vi "ProceListActMain.vi"() -> ()   [LabVIEW 2019]
uses:
  Ctrl/Right2arrow.ctl
  Ctrl/left2arrow.ctl
  Ctrl/UpLoad2.ctl
  Ctrl/Remove.ctl
  Ctrl/Up2.ctl
  Ctrl/down2.ctl
  <vilib>/Utility/miscctls.llb/LVPointTypeDef.ctl
  <vilib>/Utility/miscctls.llb/LVPositionTypeDef.ctl
  60868002-0d4d-43f0-995a-60bbf307d005.vi
  3149b30a-55dc-446c-b552-6eeb82815ac3.vi
  963f54ab-7a83-4128-af58-6966ad4c5d0f.vi
  27abb3d3-4d96-49e0-85aa-55843c44cf8e.vi
  5b1c7a0c-b8ed-4af5-97c9-577675ba5e56.vi
  577cd01a-d66b-4b05-b2ca-c7f6d430580f.vi
  87e15d9e-a7ef-48ad-a0c8-dc216d43436b.vi
  40c5cbea-e99d-4875-be97-d34c3ca007e7.vi
  <vilib>/JDP Science/JSONtext/JSON text to Variant.vi
  LLB/Commonly VI/Main Glb.vi
  Glb/ProcessListGlb.vi
  Class/Main Process Class/MPC_VirbVision/Panel RefGlb.vi
  <vilib>/JDP Science/JSONtext/Variant to JSON Text.vi
  LLB/Commonly VI.lvlib
panel:
  out "DataOutResult":string caption="輸出資料數據範例"
  out "DataOutName":string caption="輸出資料名稱"
  in  "SelectUp":T1
  in  "SelectDown":T2
  out "Action 2":string
  out "ProceListPath":path
  in  "SubUI":bool
  in  "Tab Control":enum32{"Page 1", "Page 2"}(tab)
  in  "VisionTable":i32(listbox) caption="視覺列表/VisionList"
  in  "Action":enum16{"Vision", "Virbration", "IO"}(ring)=enum."Virbration"
  in  "ProcessPage":T3(tab)=enum."None"
  in  "VisionProjectList":u16(ring) caption="專案選擇/Project Select" items=["None", "Calib", "Check", "Item1", "Item2", "Item3"]
  in  "Btn_AddVirbListAct":T4
  in  "Btn_RemoveVirbListAct":T5
  in  "VirbList":i32(listbox) caption="列表"
  in  "VirbrationProjectList":i32(listbox) caption="專案清單"
  in  "Btn_AddIOListAct":T4
  in  "Btn_RemoveIOListAct":T5
  in  "IOList":i32(listbox) caption="列表"
  in  "IOProjectList":i32(listbox) caption="專案清單"
  in  "VisionCheck":u16(ring) caption="專案選擇/Project Select" items=["None", "Calib", "Check", "Item1", "Item2", "Item3"]
  in  "ActionTable":i32(listbox) caption="動作列表/ActionList"
  in  "InsertToList":T6
  in  "UpdateActLisrVir":bool
  in  "RemoveFroimList":T7
  in  "Btn_Save":bool
  # "請選擇使用定位功能之視覺專案!!!\nPlease Select Vision Project With Location  !!!"
  # "請選擇使用Area Check演算法之視覺專案!!!\nPlease Select Vision Project With Area Check  !!!"
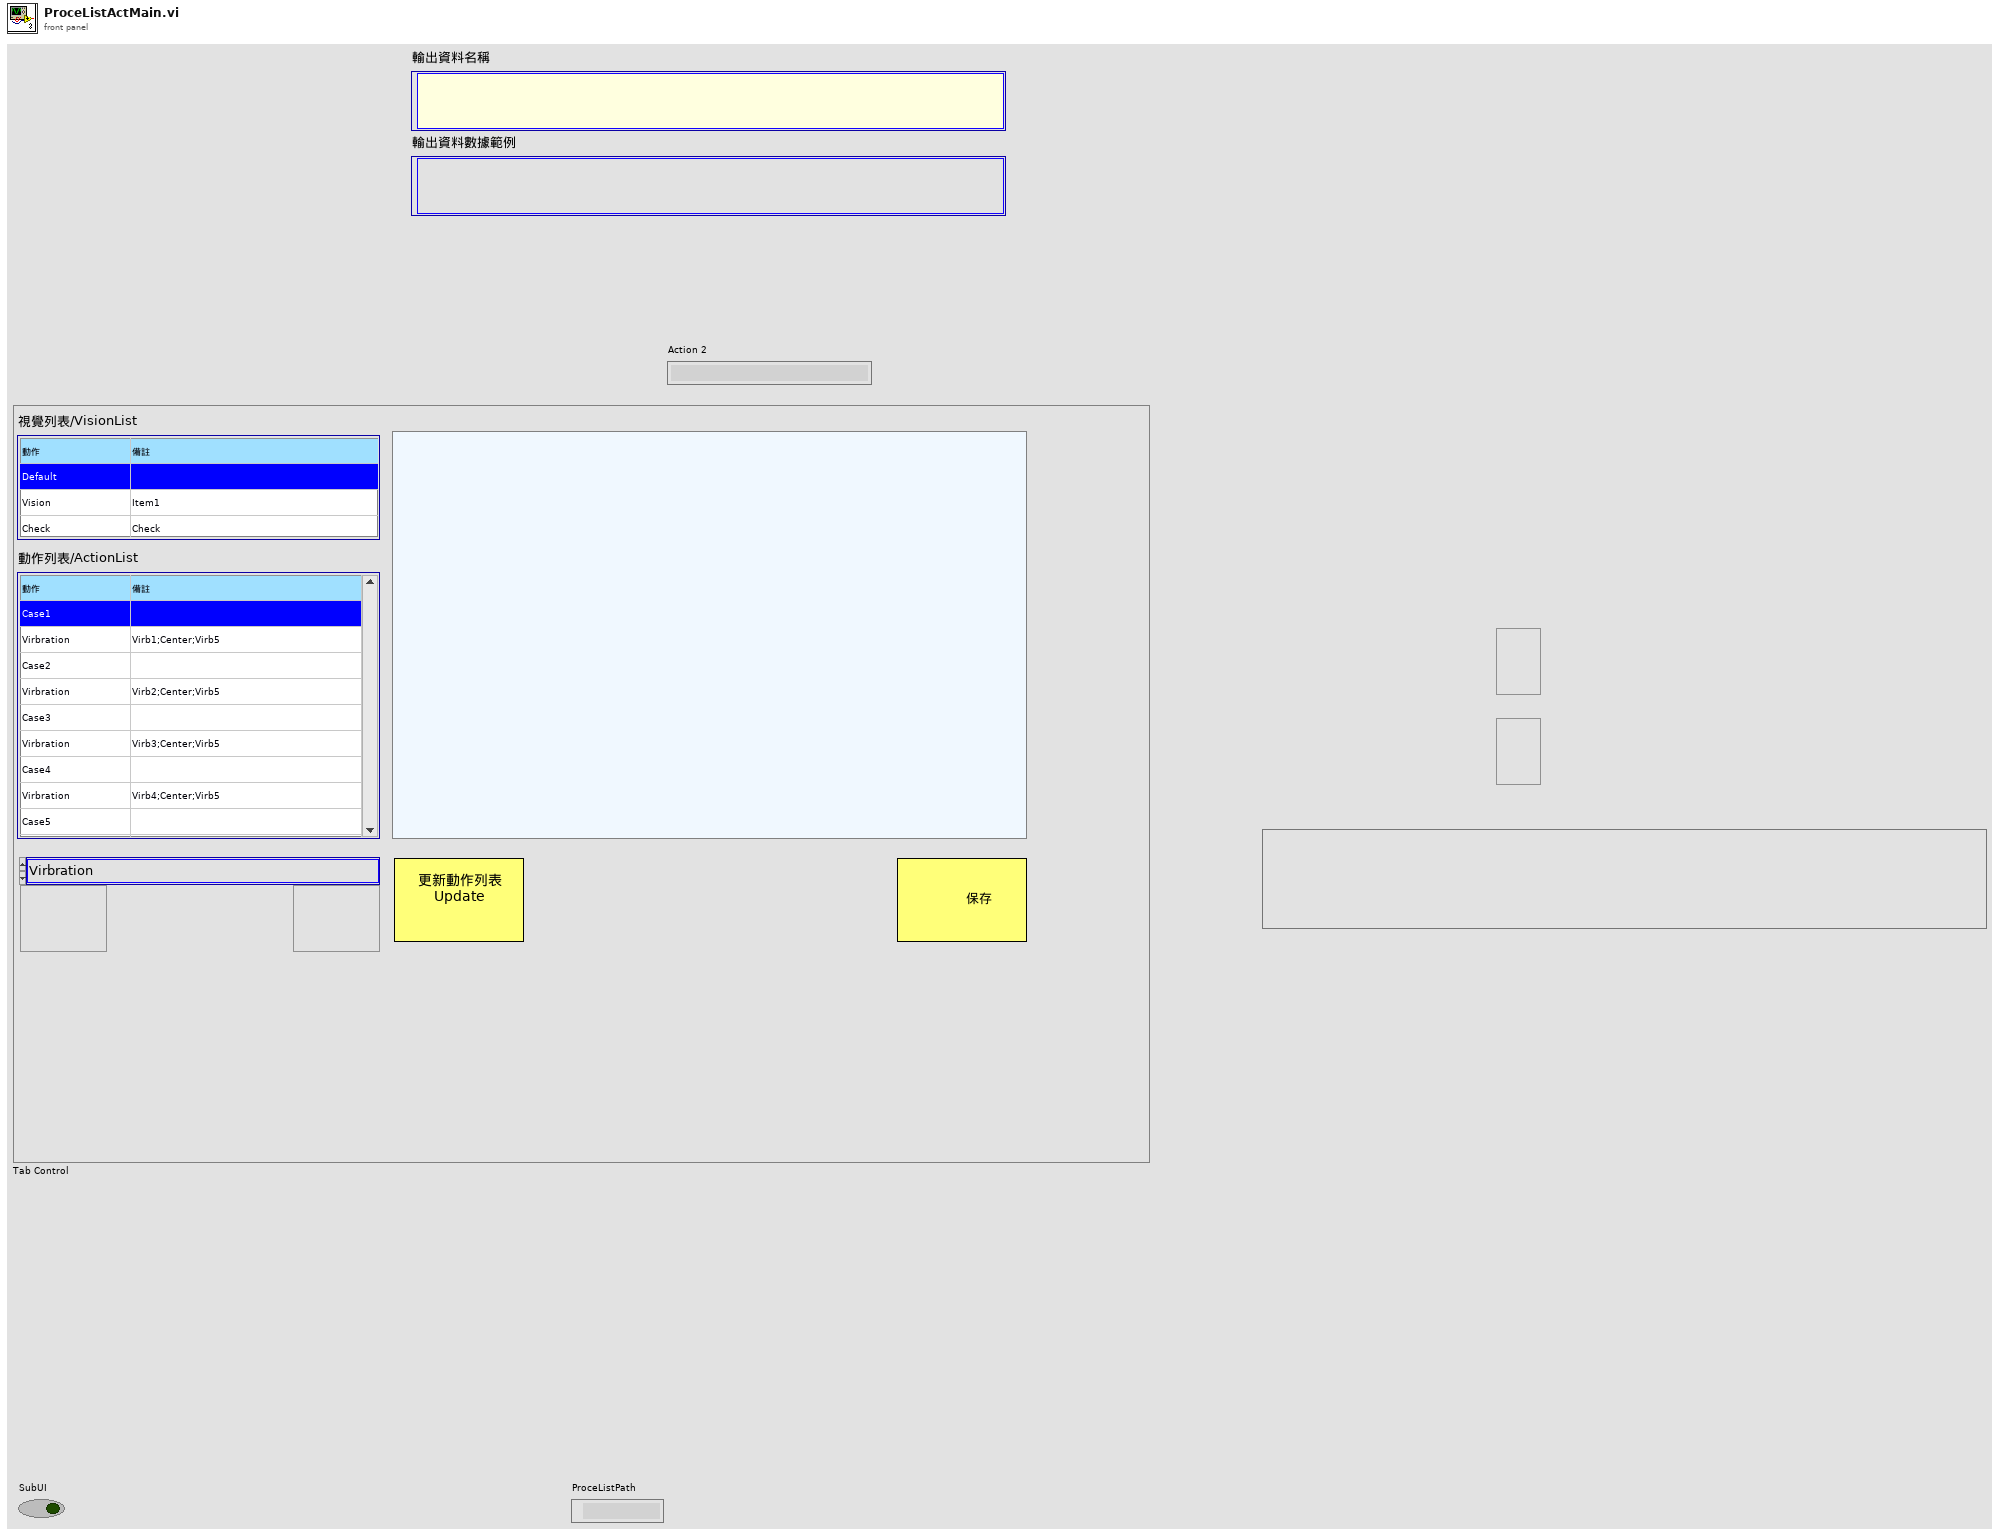
[diagram p1: front panel]
types:
  T1 = typedef "Up2.ctl" = bool
  T2 = typedef "down2.ctl" = bool
  T3 = enum32{"Vision", "Virbration", "IO", "Check", "None"}
  T4 = typedef "Right2arrow.ctl" = bool
  T5 = typedef "left2arrow.ctl" = bool
  T6 = typedef "UpLoad2.ctl" = bool
  T7 = typedef "Remove.ctl" = bool
  T8 = typedef "LVPositionTypeDef.ctl" = cluster{"Left":i32, "Top":i32}
  T9 = typedef "LVPointTypeDef.ctl" = cluster{"Horizontal":i16, "Vertical":i16}
  T10 = enum16{"Initial", "Write", "Read", "Save", "Load", "WrteAll"}
  T11 = enum16{"Initial", "Write", "Read", "Save", "Load", "Add", "Delete"}
  T12 = enum16{"initial", "write", "add", "delete", "Load", "Save", "Read", "ReadProjectName"}
  T13 = cluster{"VirbrationProjectList":refnum<vi>, "OutList":refnum<vi>}
  T14 = enum32{"invalid app kind", "Development System", "Run Time System", "Student Edition", "Embedded LabVIEW", "Evaluation", "Custom"}
  T15 = cluster{"VirbSeqName":string, "VirbSeqStep":string[]}[]
  T16 = typedef "LVPoint32TypeDef.ctl" = cluster{"Horizontal":i32, "Vertical":i32}
  T17 = cluster{"VirbrationProjectList":refnum<vi>, "VirbList":refnum<vi>}
  T18 = cluster{"IOProjectList":refnum<vi>, "IOList":refnum<vi>}
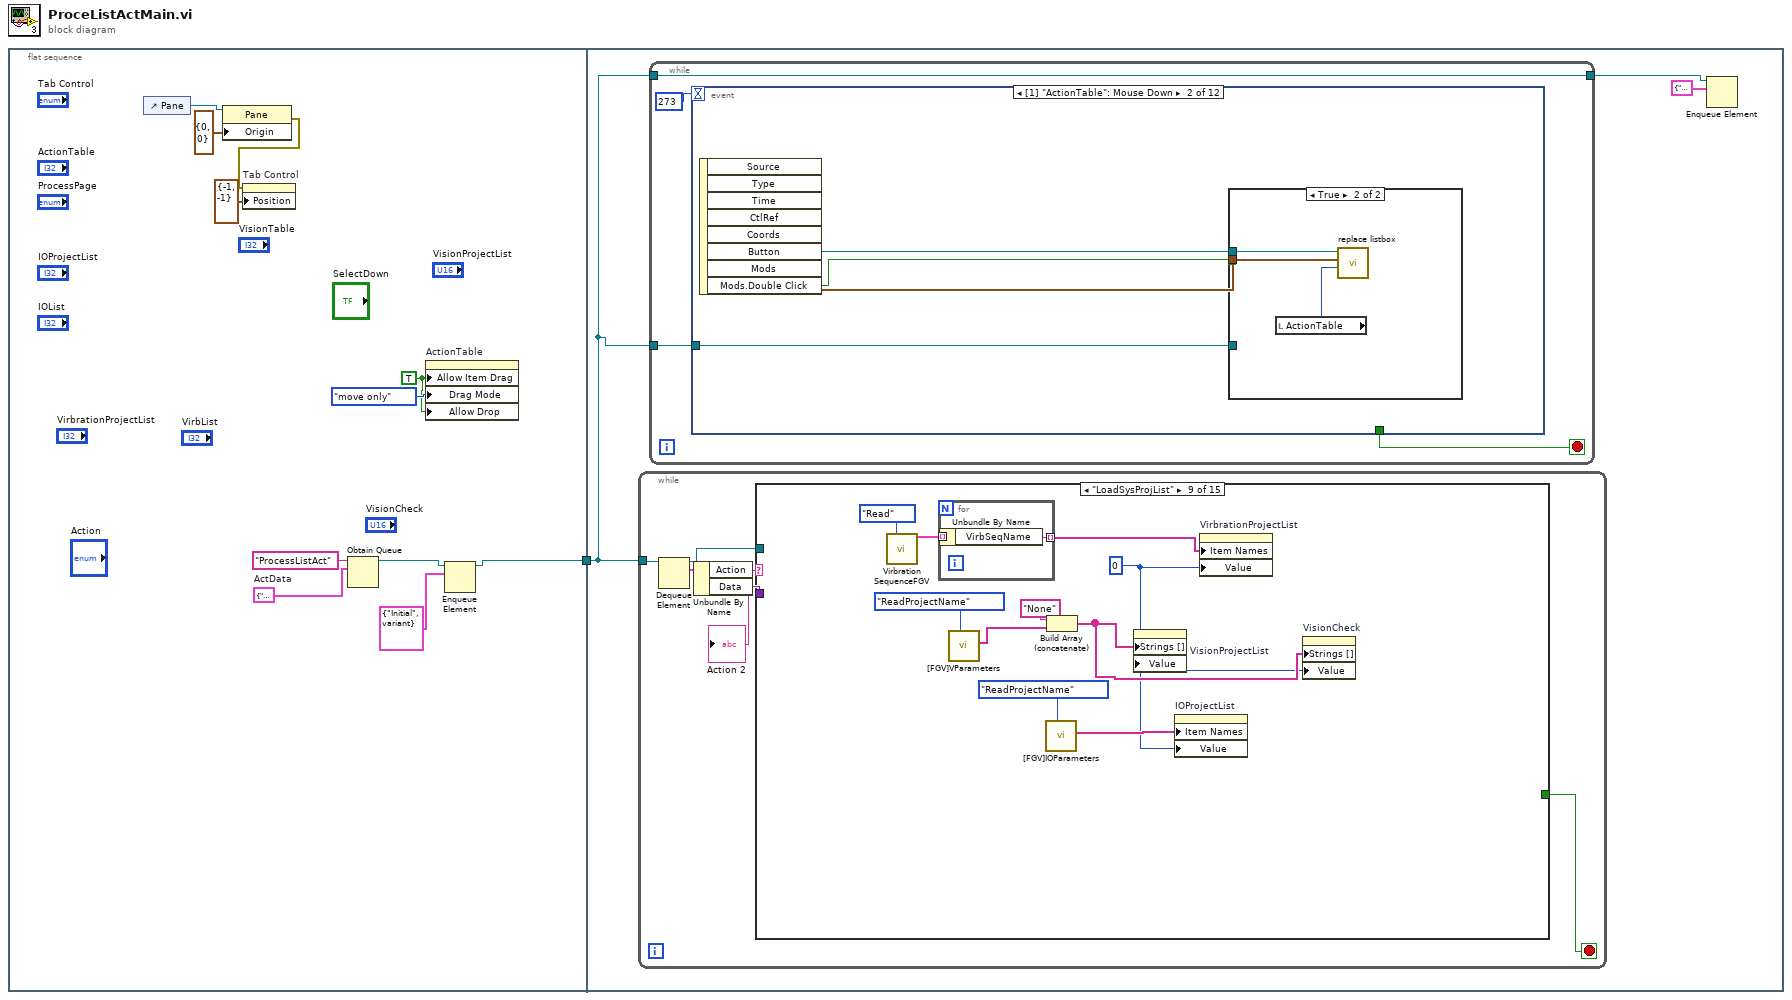
[diagram p0: block diagram]
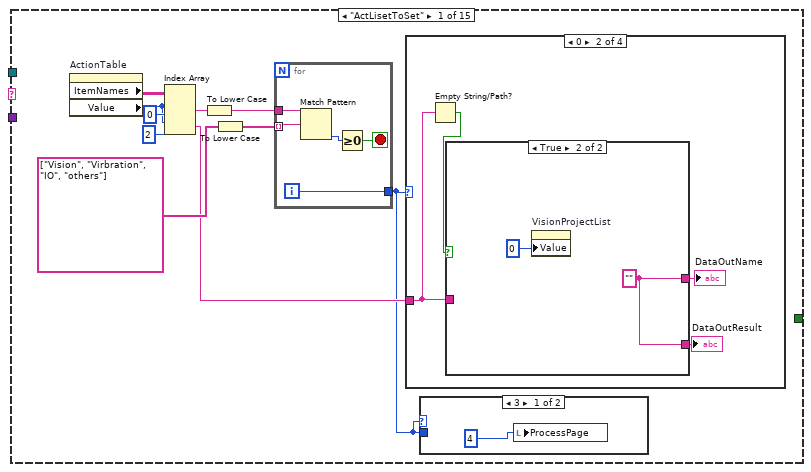
[diagram p2: hidden frame]
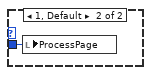
[diagram p3: hidden frame]
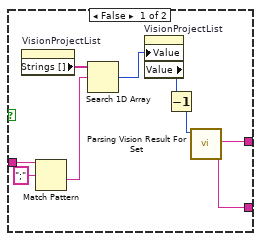
[diagram p5: hidden frame]
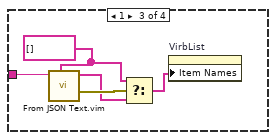
[diagram p6: hidden frame]
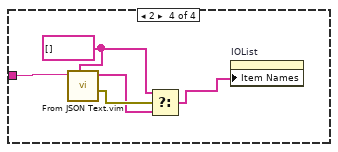
[diagram p7: hidden frame]
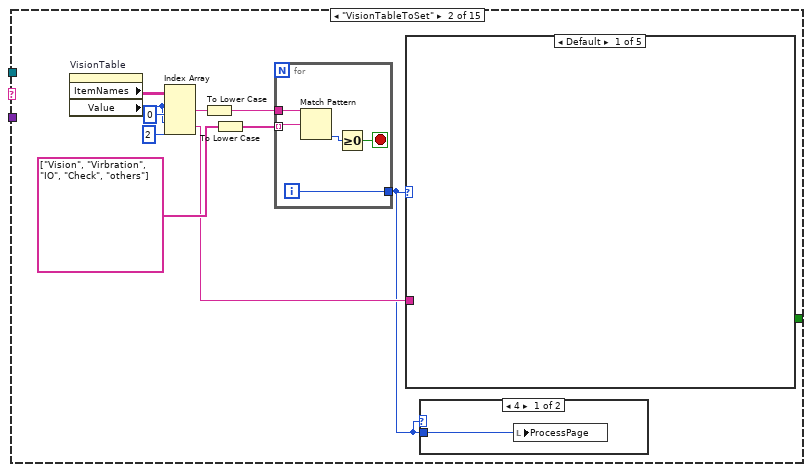
[diagram p8: hidden frame]
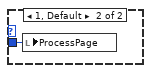
[diagram p9: hidden frame]
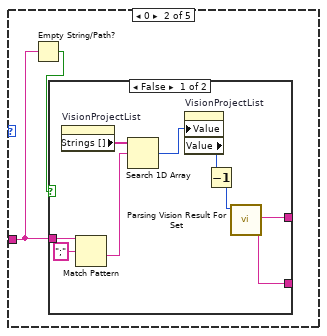
[diagram p10: hidden frame]
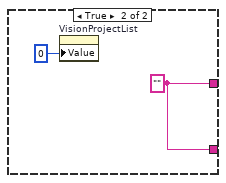
[diagram p11: hidden frame]
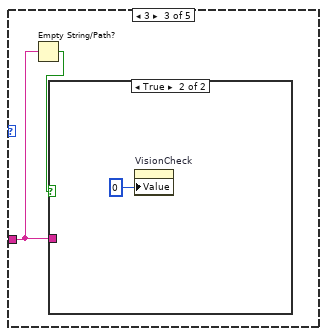
[diagram p12: hidden frame]
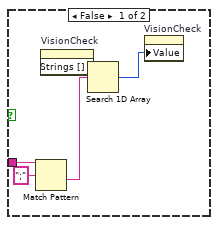
[diagram p13: hidden frame]
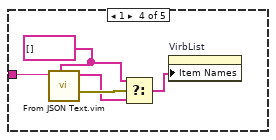
[diagram p14: hidden frame]
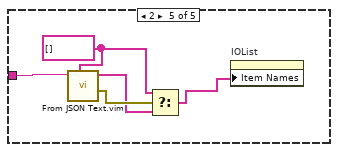
[diagram p15: hidden frame]
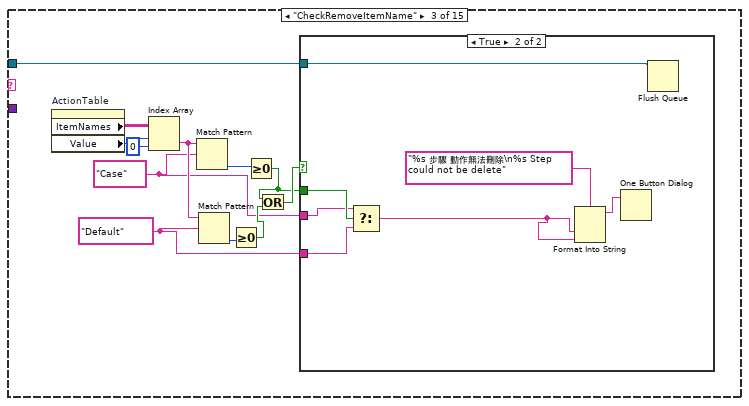
[diagram p16: hidden frame]
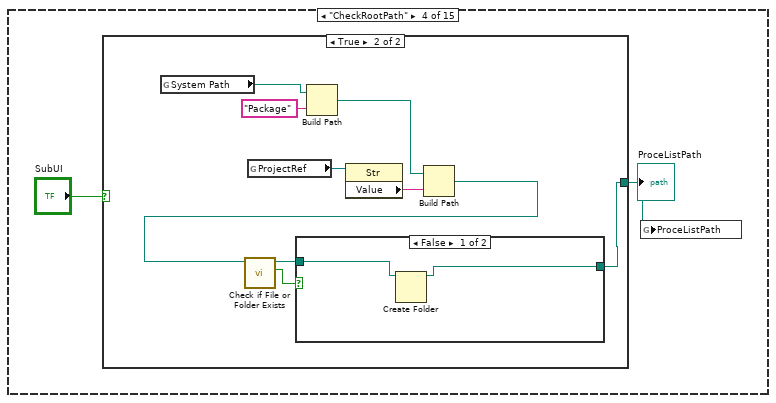
[diagram p18: hidden frame]
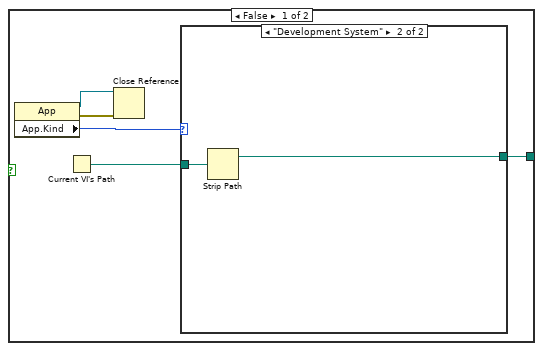
[diagram p19: hidden frame]
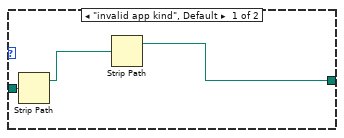
[diagram p20: hidden frame]
diagram:
  n1 = flat-sequence {
    tunnel: [w8] -> w1
    tunnel: w1 -> [w13]
    frame #0 {
      w6 = TRUE ("Drag/Drop:Allow Dragging")
      w11 = cluster{"Action":string, "Data":variant} {"Action"="", "Data"=variant}  # ActData
      n2 = control-ref of="Pane"() -> (w5:refnum<vi>)
      n3 = property class="Pane"(reference=w5, "Origin"=T9 {"Horizontal"=0, "Vertical"=0}) -> (error out=w3:errorcluster)  [unwired: 1 in, 1 out]
      n4 = property on="Tab Control" class="TabCtl (strict)"(error in=w3, "Position"=T8 {"Left"=-1, "Top"=-1}) -> ()  [unwired: 1 in, 2 out]
      n5 = Obtain Queue(name (unnamed)="ProcessListAct", element data type=w11) -> (queue out=w9:refnum<queue>)  [unwired: 3 in, 2 out]
      n6 = property on="ActionTable" class="MCListbox (strict)"("Allow Item Drag"=w6, "Drag Mode"=enum32{"copy or move", "copy only", "move only"}."move only" ("Drag/Drop:Drag Mode"), "Allow Drop"=w6) -> ()  [unwired: 2 in, 2 out]
      n7 = Enqueue Element(queue=w9, element=cluster{"Action":string, "Data":variant} {"Action"="Initial", "Data"=variant}) -> (queue out=w8:refnum<queue>)  [unwired: 2 in, 2 out]
    }
    frame #1 {
      n8 = while {
        tunnel: w13 -> [w21]
        stop <- w18 stop-if-true
        n9 = Dequeue Element(queue=w21) -> (queue out=w17:refnum<queue>, element=w20:cluster{"Action":string, "Data":variant})  [unwired: 2 in, 2 out]
        n10 = Unbundle By Name(w20) -> ("Action"=w19:string, "Data"=w16:variant)
        "Action 2" <- w19
        n11 = case shown="\"LoadSysProjList\"" w19 {
          tunnel: [_ _ _ _ _ _ _ _ _ _ _ _ _ _ w301] -> w18
          tunnel: w17 -> [_ _ w119 _ _ w158 _ _ _ _ _ _ _ _ _]
          tunnel: w16 -> [_ _ _ _ _ _ _ _ _ _ w203 _ w226 _ _]
          frame "ActLisetToSet" {
            n12 = property on="ActionTable" class="MCListbox (strict)"() -> ("ItemNames"=w31:string[][], "Value"=w25:i32)  [unwired: 2 in, 2 out]
            n13 = Index Array(array=w31, index (row) #1=w25, index (col) #1=0 ("disabled index (col)"), index (row) #2=w25, index (col) #2=2 ("disabled index (col)")) -> (element #1=w28:string, element #2=w23:string)
            n14 = To Lower Case(string=w28) -> (all lower case string=w27:string)
            n15 = To Lower Case(string=string[] ["Vision", "Virbration", "IO", "others"]) -> (all lower case string=w26:string[])
            n16 = for {
              tunnel: w26 -> [w62] mode=indexing
              tunnel: w27 -> [w63]
              tunnel: [w59] -> w22
              i -> [w59]
              stop <- w60 stop-if-true
              n17 = Match Pattern(string=w63, regular expression=w62) -> (offset past match=w61:i32)  [unwired: 1 in, 3 out]
              n18 = Greater Or Equal To 0?(x=w61) -> (x >= 0?=w60:bool)
            }
            n19 = case shown="0" w22 {
              tunnel: w23 -> [_ w35 w53 w58]
              frame Default {
              }
              frame 0 {
                n20 = Empty String/Path?(string/path=w35) -> (empty?=w34:bool)
                n21 = case shown="True" w34 {
                  tunnel: [w46 w48] -> w37
                  tunnel: [w45 w48] -> w36
                  tunnel: w35 -> [w42 _]
                  frame False {
                    n22 = property on="VisionProjectList" class="Ring (strict)"() -> ("Strings []"=w40:string[])  [unwired: 2 in, 2 out]
                    n23 = Match Pattern(string=w42, regular expression=";") -> (after substring=w38:string)  [unwired: 1 in, 3 out]
                    n24 = Search 1D Array(1D array=w40, element=w38) -> (index of element=w39:i32)  [unwired: 1 in]
                    n25 = property on="VisionProjectList" class="Ring (strict)"("Value"=w39) -> ("Value"=w44:u16)  [unwired: 2 in, 2 out]
                    n26 = Decrement(x=w44) -> (x-1=w43:u16)
                    n27 = call "Parsing Vision Result For Set.vi"("VisionProject"=w43) -> ("Dataout"=w46:string, "DataoutName"=w45:string)  [unwired: 9 in]
                  }
                  frame True {
                    w48 = "" ("DataoutName")
                    n28 = property on="VisionProjectList" class="Ring (strict)"("Value"=0) -> ()  [unwired: 2 in, 2 out]
                  }
                }
                "DataOutResult" <- w37
                "DataOutName" <- w36
              }
              frame 1 {
                w51 = string[] [] ("Item Names")
                n29 = call "From JSON Text.vim"("Data Type and Default Value"=w51, "JSON"=w53) -> ("error out"=w52:errorcluster, "Data out"=w49:string[])  [unwired: 8 in]
                n30 = Select(t=w51, s=w52, f=w49) -> (s? t:f=w50:string[])
                n31 = property on="VirbList" class="LstBox (strict)"("Item Names"=w50) -> ()  [unwired: 2 in, 2 out]
              }
              frame 2 {
                w55 = string[] [] ("Item Names")
                n32 = call "From JSON Text.vim"("Data Type and Default Value"=w55, "JSON"=w58) -> ("error out"=w57:errorcluster, "Data out"=w56:string[])  [unwired: 8 in]
                n33 = Select(t=w55, s=w57, f=w56) -> (s? t:f=w54:string[])
                n34 = property on="IOList" class="LstBox (strict)"("Item Names"=w54) -> ()  [unwired: 2 in, 2 out]
              }
            }
            n35 = case shown="3" w22 {
              tunnel: w22 -> [_ w33]
              frame 3 {
                n36 = local write "ProcessPage"(4) -> ()
              }
              frame 1, Default {
                n37 = local write "ProcessPage"(w33) -> ()
              }
            }
          }
          frame "VisionTableToSet" {
            n38 = property on="VisionTable" class="MCListbox (strict)"() -> ("ItemNames"=w73:string[][], "Value"=w67:i32)  [unwired: 2 in, 2 out]
            n39 = Index Array(array=w73, index (row) #1=w67, index (col) #1=0 ("disabled index (col)"), index (row) #2=w67, index (col) #2=2 ("disabled index (col)")) -> (element #1=w70:string, element #2=w65:string)
            n40 = To Lower Case(string=w70) -> (all lower case string=w69:string)
            n41 = To Lower Case(string=string[] ["Vision", "Virbration", "IO", "Check", "others"]) -> (all lower case string=w68:string[])
            n42 = for {
              tunnel: w68 -> [w110] mode=indexing
              tunnel: w69 -> [w111]
              tunnel: [w107] -> w64
              i -> [w107]
              stop <- w108 stop-if-true
              n43 = Match Pattern(string=w111, regular expression=w110) -> (offset past match=w109:i32)  [unwired: 1 in, 3 out]
              n44 = Greater Or Equal To 0?(x=w109) -> (x >= 0?=w108:bool)
            }
            n45 = case shown="Default" w64 {
              tunnel: w65 -> [_ w77 w90 w101 w106]
              frame Default {
              }
              frame 0 {
                n46 = Empty String/Path?(string/path=w77) -> (empty?=w76:bool)
                n47 = case shown="False" w76 {
                  tunnel: [w86 w88] -> _
                  tunnel: [w85 w88] -> _
                  tunnel: w77 -> [w82 _]
                  frame False {
                    n48 = property on="VisionProjectList" class="Ring (strict)"() -> ("Strings []"=w80:string[])  [unwired: 2 in, 2 out]
                    n49 = Match Pattern(string=w82, regular expression=";") -> (after substring=w78:string)  [unwired: 1 in, 3 out]
                    n50 = Search 1D Array(1D array=w80, element=w78) -> (index of element=w79:i32)  [unwired: 1 in]
                    n51 = property on="VisionProjectList" class="Ring (strict)"("Value"=w79) -> ("Value"=w84:u16)  [unwired: 2 in, 2 out]
                    n52 = Decrement(x=w84) -> (x-1=w83:u16)
                    n53 = call "Parsing Vision Result For Set.vi"("VisionProject"=w83) -> ("Dataout"=w86:string, "DataoutName"=w85:string)  [unwired: 9 in]
                  }
                  frame True {
                    w88 = "" ("DataoutName")
                    n54 = property on="VisionProjectList" class="Ring (strict)"("Value"=0) -> ()  [unwired: 2 in, 2 out]
                  }
                }
              }
              frame 3 {
                n55 = Empty String/Path?(string/path=w90) -> (empty?=w89:bool)
                n56 = case shown="True" w89 {
                  tunnel: w90 -> [w95 _]
                  frame False {
                    n57 = Match Pattern(string=w95, regular expression=";") -> (after substring=w91:string)  [unwired: 1 in, 3 out]
                    n58 = property on="VisionCheck" class="Ring (strict)"() -> ("Strings []"=w93:string[])  [unwired: 2 in, 2 out]
                    n59 = Search 1D Array(1D array=w93, element=w91) -> (index of element=w92:i32)  [unwired: 1 in]
                    n60 = property on="VisionCheck" class="Ring (strict)"("Value"=w92) -> ()  [unwired: 2 in, 2 out]
                  }
                  frame True {
                    n61 = property on="VisionCheck" class="Ring (strict)"("Value"=0) -> ()  [unwired: 2 in, 2 out]
                  }
                }
              }
              frame 1 {
                w99 = string[] [] ("Item Names")
                n62 = call "From JSON Text.vim"("Data Type and Default Value"=w99, "JSON"=w101) -> ("error out"=w100:errorcluster, "Data out"=w97:string[])  [unwired: 8 in]
                n63 = Select(t=w99, s=w100, f=w97) -> (s? t:f=w98:string[])
                n64 = property on="VirbList" class="LstBox (strict)"("Item Names"=w98) -> ()  [unwired: 2 in, 2 out]
              }
              frame 2 {
                w103 = string[] [] ("Item Names")
                n65 = call "From JSON Text.vim"("Data Type and Default Value"=w103, "JSON"=w106) -> ("error out"=w105:errorcluster, "Data out"=w104:string[])  [unwired: 8 in]
                n66 = Select(t=w103, s=w105, f=w104) -> (s? t:f=w102:string[])
                n67 = property on="IOList" class="LstBox (strict)"("Item Names"=w102) -> ()  [unwired: 2 in, 2 out]
              }
            }
            n68 = case shown="4" w64 {
              tunnel: w64 -> [w74 w75]
              frame 4 {
                n69 = local write "ProcessPage"(w74) -> ()
              }
              frame 1, Default {
                n70 = local write "ProcessPage"(w75) -> ()
              }
            }
          }
          frame "CheckRemoveItemName" {
            w112 = "Default" ("regular expression")
            w113 = "Case" ("regular expression")
            n71 = property on="ActionTable" class="MCListbox (strict)"() -> ("ItemNames"=w123:string[][], "Value"=w122:i32)  [unwired: 2 in, 2 out]
            n72 = Index Array(array=w123, index (row)=w122, index (col)=0 ("disabled index (col)")) -> (element=w117:string)
            n73 = Match Pattern(string=w117, regular expression=w113) -> (offset past match=w120:i32)  [unwired: 1 in, 3 out]
            n74 = Match Pattern(string=w117, regular expression=w112) -> (offset past match=w116:i32)  [unwired: 1 in, 3 out]
            n75 = Greater Or Equal To 0?(x=w116) -> (x >= 0?=w115:bool)
            n76 = Greater Or Equal To 0?(x=w120) -> (x >= 0?=w114:bool)
            n77 = Or(x=w114, y=w115) -> (x .or. y?=w118:bool)
            n78 = case shown="True" w118 {
              tunnel: w119 -> [_ w130]
              tunnel: w114 -> [_ w129]
              tunnel: w113 -> [_ w128]
              tunnel: w112 -> [_ w127]
              frame False {
              }
              frame True {
                n79 = Select(t=w128, s=w129, f=w127) -> (s? t:f=w125:string)
                n80 = Format Into String(format string="%s 步驟 動作無法刪除\n%s Step could not be delete" ("message"), w125, w125) -> (resulting string=w124:string)  [unwired: 2 in, 1 out]
                n81 = One Button Dialog(message=w124) -> ()  [unwired: 1 in, 1 out]
                n82 = Flush Queue(queue=w130) -> ()  [unwired: 1 in, 3 out]
              }
            }
          }
          frame "CheckRootPath" {
            n83 = case shown="True" "SubUI" {
              tunnel: [w133 w145] -> w131
              frame False {
                n84 = property class="App"() -> (reference out=w134:refnum<vi>, error out=w135:errorcluster, "App.Kind"=w137:T14)  [unwired: 2 in]
                n85 = Current VI's Path() -> (path=w136:path)
                n86 = Close Reference(reference=w134, error in (no error)=w135) -> ()  [unwired: 1 out]
                n87 = case shown="\"Development System\"" w137 {
                  tunnel: w136 -> [w140 w142]
                  tunnel: [w138 w141] -> w133
                  frame "invalid app kind", Default {
                    n88 = Strip Path(path=w140) -> (stripped path=w139:path)  [unwired: 1 out]
                    n89 = Strip Path(path=w139) -> (stripped path=w138:path)  [unwired: 1 out]
                  }
                  frame "Development System" {
                    n90 = Strip Path(path=w142) -> (stripped path=w141:path)  [unwired: 1 out]
                  }
                }
              }
              frame True {
                n91 = global read "Main Glb.vi" "System Path"() -> (w149:path)
                n92 = global read "Main Glb.vi" "ProjectRef"() -> (w151:refnum<vi>)
                n93 = Build Path(base path=w149, name or relative path="Package") -> (appended path=w148:path)
                n94 = property class="Str"(reference=w151) -> ("Value"=w150:string)  [unwired: 1 in, 2 out]
                n95 = Build Path(base path=w148, name or relative path=w150) -> (appended path=w143:path)
                n96 = call <vilib>:"Check if File or Folder Exists.vi"("path"=w143) -> ("file or folder exists?"=w146:bool, "dup path"=w144:path)  [unwired: 8 in, 1 out]
                n97 = case shown="False" w146 {
                  tunnel: [w152 w154] -> w145
                  tunnel: w144 -> [w153 w154]
                  frame False {
                    n98 = Create Folder(path (use dialog)=w153) -> (created path=w152:path)  [unwired: 2 in, 2 out]
                  }
                  frame True {
                  }
                }
              }
            }
            "ProceListPath" <- w131
            n99 = global write "ProcessListGlb.vi" "ProceListPath"(w131) -> ()
          }
          frame "False", Default {
          }
          frame "Initial" {
            w161 = string[] [] ("Item Names")
            n100 = control-ref of="This VI"() -> (w157:refnum<vi>)
            n101 = invoke class="VI" method="Default Vals.Reinit All"(reference=w157) -> ()  [unwired: 2 in, 3 out]
            n102 = for {
              tunnel: w158 -> [w163]
              tunnel: cluster{"Action":string, "Data":variant}[] [{"Action"="CheckRootPath", "Data"=variant}, {"Action"="LoadProject", "Data"=variant}, {"Action"="LoadSysProjList", "Data"=variant}, {"Action"="loadfinish", "Data"=variant}] -> [w162] mode=indexing
              n103 = Enqueue Element(queue=w163, element=w162) -> ()  [unwired: 2 in, 3 out]
            }
            n104 = property on="VirbrationProjectList" class="LstBox (strict)"("Item Names"=w161) -> ()  [unwired: 2 in, 2 out]
            n105 = property on="IOList" class="LstBox (strict)"("Item Names"=w161) -> ()  [unwired: 2 in, 2 out]
            n106 = property on="VirbList" class="LstBox (strict)"("Item Names"=w161) -> ()  [unwired: 2 in, 2 out]
            n107 = property on="IOProjectList" class="LstBox (strict)"("Item Names"=w161) -> ()  [unwired: 2 in, 2 out]
            n108 = local write "ProcessPage"(T3."None" ("ProcessPage")) -> ()
            n109 = property on="VisionTable" class="MCListbox (strict)"("ItemNames"=string[][] [["Default", "", "", "0"], ["Vision", "", "", "1"], ["Check", "", "", "2"], ["", "", "", ""], ["", "", "", ""], ["", "", "", ""], ["", "", "", ""], ["", "", "", ""], ["", "", "", ""], ["", "", "", ""], ["", "", "", ""], ["", "", "", ""], ["", "", "", ""], ["22", "", "", ""], ["23", "", "", ""], ["24", "", "", ""], ["25", "", "", ""]] ("Item Names")) -> ()  [unwired: 2 in, 2 out]
            n110 = property on="ActionTable" class="MCListbox (strict)"("ItemNames"=string[][] [["Case1", "", "", "1"], ["Case2", "", "", "2"], ["Case3", "", "", "3"], ["Case4", "", "", "4"], ["Case5", "", "", "5"], ["Case6", "", "", "6"], ["Case7", "", "", "7"], ["Case8", "", "", "8"], ["Case9", "", "", "9"], ["Case10", "", "", "10"], ["", "", "", ""], ["", "", "", ""], ["", "", "", ""], ["", "", "", ""], ["", "", "", ""], ["", "", "", ""], ["", "", "", ""], ["", "", "", ""], ["", "", "", ""], ["", "", "", ""], ["22", "", "", ""], ["23", "", "", ""], ["24", "", "", ""], ["25", "", "", ""]] ("Item Names")) -> ()  [unwired: 2 in, 2 out]
          }
          frame "InsertToList" {
            w167 = ""
            n111 = property on="ActionTable" class="MCListbox (strict)"() -> ("ItemNames"=w170:string[][], "Value"=w164:i32)  [unwired: 2 in, 2 out]
            n112 = property on="Action" class="Enum (strict)"() -> ("RingText.Text"=w168:string)  [unwired: 2 in, 2 out]
            n113 = Build Array(w168, w167, w167, "-1") -> (w165:string[])
            n114 = Insert Into Array(array=w170, index (row)=w164, new element=w165) -> (w169:string[][])  [unwired: 1 in]
            n115 = property on="ActionTable" class="MCListbox (strict)"("ItemNames"=w169) -> ()  [unwired: 2 in, 2 out]
          }
          frame "LoadProject" {
            n116 = call "Process List FGV.vi"("Action"=T10."Load") -> ("TableOut"=w175:string[][])  [unwired: 12 in, 2 out]
            n117 = Delete From Array(array=w175, length=3, index (row)=0) -> (deleted portion=w171:string[][], array with subset deleted=w172:string[][])  [unwired: 1 in]
            n118 = property on="ActionTable" class="MCListbox (strict)"("ItemNames"=w172) -> (error out=w176:errorcluster)  [unwired: 2 in, 1 out]
            n119 = property on="VisionTable" class="MCListbox (strict)"("ItemNames"=w171) -> ()  [unwired: 2 in, 2 out]
            n120 = call "Request UI.vi"("error in (no error)"=w176, "Data"=cluster{"Action":string, "Data":variant} {"Action"="ProjectToUI", "Data"=variant}) -> ()  [unwired: 8 in, 2 out]
          }
          frame "LoadSysProjList" {
            w182 = 0 ("VirbrationProjectList")
            n121 = call "Virbration SequenceFGV.vi"("Action"=T11."Read") -> ("VirbSeqDataList"=w180:T15)  [unwired: 12 in, 2 out]
            n122 = for {
              tunnel: w180 -> [w190] mode=indexing
              tunnel: [w189] -> w179 mode=indexing
              n123 = Unbundle By Name(w190) -> ("VirbSeqName"=w189:string)
            }
            n124 = call "[FGV]VParameters.vi"("Enum"=T12."ReadProjectName") -> ("ProjectName"=w185:string[])  [unwired: 7 in, 3 out]
            n125 = call "[FGV]IOParameters.vi"("Enum"=T12."ReadProjectName") -> ("ProjectName"=w187:string[])  [unwired: 8 in, 2 out]
            n126 = Build Array (concatenate)("None", w185) -> (w183:string[])
            n127 = property on="VisionProjectList" class="Ring (strict)"("Strings []"=w183, "Value"=w182) -> ()  [unwired: 2 in, 2 out]
            n128 = property on="IOProjectList" class="LstBox (strict)"("Item Names"=w187, "Value"=w182) -> ()  [unwired: 2 in, 2 out]
            n129 = property on="VirbrationProjectList" class="LstBox (strict)"("Item Names"=w179, "Value"=w182) -> ()  [unwired: 2 in, 2 out]
            n130 = property on="VisionCheck" class="Ring (strict)"("Strings []"=w183, "Value"=w182) -> ()  [unwired: 2 in, 2 out]
          }
          frame "loadfinish" {
            n131 = global write "Panel RefGlb.vi" "Process load"(TRUE ("Process load")) -> ()
          }
          frame "ProjListToActList" {
            n132 = Variant To Data(type=T13 {"VirbrationProjectList"=refnum, "OutList"=refnum}, Variant=w203) -> (data=w198:T13, error out=w202:errorcluster)  [unwired: 1 in]
            n133 = Unbundle(w198) -> ("VirbrationProjectList"=w197:refnum<vi>, "OutList"=w196:refnum<vi>)
            n134 = property class="LstBox (strict)"(reference=w197, error in=w202) -> ("Item Names"=w201:string[], "Value"=w200:i32)  [unwired: 2 out]
            n135 = Index Array(array=w201, index=w200) -> (element=w194:string)
            n136 = property class="LstBox (strict)" props=["Item Names", "Value"](reference=w196) -> (reference out=w193:refnum<vi>, "Item Names"=w195:string[])  [unwired: 1 in, 2 out]
            n137 = Build Array (concatenate)(w195, w194) -> (w192:string[])
            n138 = property class="LstBox (strict)"(reference=w193, "Item Names"=w192) -> ()  [unwired: 1 in, 2 out]
          }
          frame "RemoveFroimList" {
            n139 = property on="ActionTable" class="MCListbox (strict)"() -> ("ItemNames"=w207:string[][], "Value"=w204:i32)  [unwired: 2 in, 2 out]
            n140 = Index Array(array=w207, index (row) #1=w204, index (col) #1=0 ("disabled index (col)"), index (row) #2=w204, index (col) #2=1 ("disabled index (col)")) -> (element #1=w206:string, element #2=w205:string)
            n141 = Format Into String(format string="確認是否移除步驟%s , %s\nCheck Delete Step %s , %s", w206, w205, w206, w205) -> (resulting string=w209:string)  [unwired: 2 in, 1 out]
            n142 = Two Button Dialog(message=w209) -> (T button?=w208:bool)  [unwired: 2 in]
            n143 = case shown="True" w208 {
              tunnel: w207 -> [_ w216]
              tunnel: w204 -> [_ w213]
              frame False {
              }
              frame True {
                n144 = Delete From Array(array=w216, length=1, index (row)=w213) -> (array with subset deleted=w215:string[][])  [unwired: 1 in, 1 out]
                n145 = property on="ActionTable" class="MCListbox (strict)"("ItemNames"=w215) -> ()  [unwired: 2 in, 2 out]
              }
            }
          }
          frame "RemoveListAct" {
            n146 = Variant To Data(type=T13 {"VirbrationProjectList"=refnum, "OutList"=refnum}, Variant=w226) -> (data=w224:T13)  [unwired: 1 in, 1 out]
            n147 = Unbundle(w224) -> ("OutList"=w223:refnum<vi>)  [unwired: 1 out]
            n148 = property class="LstBox (strict)"(reference=w223) -> (reference out=w221:refnum<vi>, "Item Names"=w222:string[], "Value"=w219:i32)  [unwired: 1 in, 1 out]
            n149 = Delete From Array(array=w222, length=1, index=w219) -> (array with subset deleted=w218:string[])  [unwired: 1 out]
            n150 = property class="LstBox (strict)"(reference=w221, "Item Names"=w218, "Value"=0) -> ()  [unwired: 1 in, 2 out]
          }
          frame "SetToActlist" {
            n151 = local read "ProcessPage"() -> (w227:T3)
            n152 = case shown="Default" w227 {
              tunnel: w227 -> [_ w236 w268]
              frame Default {
              }
              frame "Virbration" {
                n153 = case shown="\"Virbration\"" w236 {
                  tunnel: [w240 w252 w259] -> w233
                  tunnel: [w237 w246 w254] -> w229
                  frame "Vision", Default {
                    n154 = property on="VisionProjectList" class="Ring (strict)"() -> (error out=w243:errorcluster, "Value"=w245:u16, "RingText.Text"=w237:string)  [unwired: 2 in, 1 out]
                    n155 = Decrement(x=w245) -> (x-1=w244:u16)
                    n156 = Number To Decimal String(number=w244) -> (decimal integer string=w239:string)  [unwired: 1 in]
                    n157 = property on="VisionProjectList" class="Ring (strict)"(error in=w243, "Value"=0) -> (error out=w241:errorcluster)  [unwired: 1 in, 1 out]
                    n158 = invoke on="DataOutResult" class="Str" method="Reinit To Default"(error in=w241) -> ()  [unwired: 2 in, 3 out]
                    n159 = invoke on="DataOutName" class="Str" method="Reinit To Default"(error in=w241) -> ()  [unwired: 2 in, 3 out]
                    n160 = Concatenate Strings(w239, ";" ("string"), w237) -> (w240:string)
                  }
                  frame "Virbration" {
                    n161 = property on="VirbList" class="LstBox (strict)"() -> (error out=w251:errorcluster, "Item Names"=w249:string[])  [unwired: 2 in, 1 out]
                    n162 = call "To JSON Text.vim"("Anything"=w249) -> ("<JSON>"=w252:string)  [unwired: 9 in, 1 out]
                    n163 = property on="VirbList" class="LstBox (strict)"(error in=w251, "Item Names"=string[] []) -> ()  [unwired: 1 in, 2 out]
                    n164 = Array To Spreadsheet String(delimiter (Tab)=";", array=w249, 3:"%s" ("format string")) -> (spreadsheet string=w246:string)
                  }
                  frame "IO" {
                    n165 = property on="IOList" class="LstBox (strict)"() -> (error out=w258:errorcluster, "Item Names"=w253:string[])  [unwired: 2 in, 1 out]
                    n166 = call "To JSON Text.vim"("Anything"=w253) -> ("<JSON>"=w259:string)  [unwired: 9 in, 1 out]
                    n167 = property on="IOList" class="LstBox (strict)"(error in=w258, "Item Names"=string[] []) -> ()  [unwired: 1 in, 2 out]
                    n168 = Array To Spreadsheet String(delimiter (Tab)=";", array=w253, 3:"%s" ("format string")) -> (spreadsheet string=w254:string)
                  }
                }
                n169 = property on="ActionTable" class="MCListbox (strict)"() -> ("ItemNames"=w234:string[][], "Value"=w231:i32)  [unwired: 2 in, 2 out]
                n170 = call <vilib>:"Trim Whitespace.vi"("string"=w229) -> ("trimmed string"=w228:string)  [unwired: 1 in]
                n171 = Replace Array Subset(array=w234, new element #1=w233, index (row) #1=w231, index (col) #1=2 ("disabled index (col)"), new element #2=w228, index (row) #2=w231, index (col) #2=1 ("disabled index (col)")) -> (w235:string[][])
                n172 = property on="ActionTable" class="MCListbox (strict)"("ItemNames"=w235) -> ()  [unwired: 2 in, 2 out]
              }
              frame "Vision", "Check" {
                n173 = case shown="\"Check\"" w268 {
                  tunnel: [w272 w281 w293 w300] -> w265
                  tunnel: [w269 w278 w287 w295] -> w261
                  frame "Vision", Default {
                    n174 = property on="VisionProjectList" class="Ring (strict)"() -> (error out=w275:errorcluster, "Value"=w277:u16, "RingText.Text"=w269:string)  [unwired: 2 in, 1 out]
                    n175 = Decrement(x=w277) -> (x-1=w276:u16)
                    n176 = Number To Decimal String(number=w276) -> (decimal integer string=w271:string)  [unwired: 1 in]
                    n177 = property on="VisionProjectList" class="Ring (strict)"(error in=w275, "Value"=0) -> (error out=w273:errorcluster)  [unwired: 1 in, 1 out]
                    n178 = invoke on="DataOutResult" class="Str" method="Reinit To Default"(error in=w273) -> ()  [unwired: 2 in, 3 out]
                    n179 = invoke on="DataOutName" class="Str" method="Reinit To Default"(error in=w273) -> ()  [unwired: 2 in, 3 out]
                    n180 = Concatenate Strings(w271, ";" ("string"), w269) -> (w272:string)
                  }
                  frame "Check" {
                    n181 = property on="VisionCheck" class="Ring (strict)"() -> (error out=w284:errorcluster, "Value"=w286:u16, "RingText.Text"=w278:string)  [unwired: 2 in, 1 out]
                    n182 = Decrement(x=w286) -> (x-1=w285:u16)
                    n183 = Number To Decimal String(number=w285) -> (decimal integer string=w280:string)  [unwired: 1 in]
                    n184 = property on="VisionCheck" class="Ring (strict)"(error in=w284, "Value"=0) -> (error out=w282:errorcluster)  [unwired: 1 in, 1 out]
                    n185 = invoke on="DataOutResult" class="Str" method="Reinit To Default"(error in=w282) -> ()  [unwired: 2 in, 3 out]
                    n186 = invoke on="DataOutName" class="Str" method="Reinit To Default"(error in=w282) -> ()  [unwired: 2 in, 3 out]
                    n187 = Concatenate Strings(w280, ";" ("string"), w278) -> (w281:string)
                  }
                  frame "Virbration" {
                    n188 = property on="VirbList" class="LstBox (strict)"() -> (error out=w292:errorcluster, "Item Names"=w290:string[])  [unwired: 2 in, 1 out]
                    n189 = call "To JSON Text.vim"("Anything"=w290) -> ("<JSON>"=w293:string)  [unwired: 9 in, 1 out]
                    n190 = property on="VirbList" class="LstBox (strict)"(error in=w292, "Item Names"=string[] []) -> ()  [unwired: 1 in, 2 out]
                    n191 = Array To Spreadsheet String(delimiter (Tab)=";", array=w290, 3:"%s" ("format string")) -> (spreadsheet string=w287:string)
                  }
                  frame "IO" {
                    n192 = property on="IOList" class="LstBox (strict)"() -> (error out=w299:errorcluster, "Item Names"=w294:string[])  [unwired: 2 in, 1 out]
                    n193 = call "To JSON Text.vim"("Anything"=w294) -> ("<JSON>"=w300:string)  [unwired: 9 in, 1 out]
                    n194 = property on="IOList" class="LstBox (strict)"(error in=w299, "Item Names"=string[] []) -> ()  [unwired: 1 in, 2 out]
                    n195 = Array To Spreadsheet String(delimiter (Tab)=";", array=w294, 3:"%s" ("format string")) -> (spreadsheet string=w295:string)
                  }
                }
                n196 = property on="VisionTable" class="MCListbox (strict)"() -> ("ItemNames"=w266:string[][], "Value"=w263:i32)  [unwired: 2 in, 2 out]
                n197 = call <vilib>:"Trim Whitespace.vi"("string"=w261) -> ("trimmed string"=w260:string)  [unwired: 1 in]
                n198 = Replace Array Subset(array=w266, new element #1=w265, index (row) #1=w263, index (col) #1=2 ("disabled index (col)"), new element #2=w260, index (row) #2=w263, index (col) #2=1 ("disabled index (col)")) -> (w267:string[][])
                n199 = property on="VisionTable" class="MCListbox (strict)"("ItemNames"=w267) -> ()  [unwired: 2 in, 2 out]
              }
            }
          }
          frame "exit" {
            n200 = call "Exit.vi"() -> ("ExitOut"=w301:bool)  [unwired: 11 in]
          }
        }
      }
      n201 = while {
        tunnel: [w303] -> w15
        tunnel: w13 -> [w303]
        tunnel: w13 -> [w302]
        stop <- w305 stop-if-true
        n202 = event shown="[1] \"ActionTable\": Mouse Down" {
          selector: _ -> [_ _ _ _ _ _ _ _ _ _ _ _]
          dyn-events: _ -> [_ _ _ _ _ _ _ _ _ _ _ _]
          timeout: 273 -> [_ _ _ _ _ _ _ _ _ _ _ _]
          tunnel: [w306 _ _ _ _ _ _ _ _ _ _ _] -> w305
          tunnel: w302 -> [_ w307 w316 w326 w350 _ w381 w383 _ _ _ w391]
          event Timeout {
            n203 = event-data() -> ()  [unwired: 1 in, 3 out]
            n204 = call "Exit.vi"() -> ("ExitOut"=w306:bool)  [unwired: 11 in]
          }
          event "ActionTable": Mouse Down {
            n205 = event-data() -> ("CtlRef"=w309:refnum<vi>, "Coords"=w310:T16, "Mods.Double Click"=w308:bool)  [unwired: 1 in, 5 out]
            n206 = case shown="True" w308 {
              tunnel: w310 -> [_ w313]
              tunnel: w309 -> [_ w315]
              tunnel: w307 -> [w312 _]
              frame False {
                n207 = Enqueue Element(queue=w312, element=cluster{"Action":string, "Data":variant} {"Action"="ActLisetToSet", "Data"=variant}) -> ()  [unwired: 2 in, 3 out]
              }
              frame True {
                n208 = local read "ActionTable"() -> (w314:i32)
                n209 = call "replace listbox.vi"("Row"=w314, "Coords"=w313, "Listbox in"=w315) -> ()  [unwired: 9 in]
              }
            }
          }
          event "VisionTable": Mouse Down {
            n210 = event-data() -> ("CtlRef"=w318:refnum<vi>, "Coords"=w319:T16, "Mods.Double Click"=w317:bool)  [unwired: 1 in, 5 out]
            n211 = case shown="False" w317 {
              tunnel: w319 -> [_ w324]
              tunnel: w318 -> [_ w323]
              tunnel: w316 -> [w321 _]
              frame False {
                n212 = Enqueue Element(queue=w321, element=cluster{"Action":string, "Data":variant} {"Action"="VisionTableToSet", "Data"=variant}) -> ()  [unwired: 2 in, 3 out]
              }
              frame True {
                n213 = local read "VisionTable"() -> (w322:i32)
                n214 = call "replace listbox.vi"("Row"=w322, "Coords"=w324, "Listbox in"=w323) -> ()  [unwired: 9 in]
              }
            }
          }
          event Value Change {
            n215 = event-data() -> ("CtlRef"=w330:refnum<vi>)  [unwired: 1 in, 5 out]
            n216 = property class="Bool"(reference=w330) -> ("Label.Text"=w329:string)  [unwired: 1 in, 2 out]
            n217 = for {
              tunnel: w329 -> [w347]
              tunnel: string[] ["Virb", "IO", "None"] -> [w346] mode=indexing
              tunnel: [w343] -> w327
              i -> [w343]
              stop <- w344 stop-if-true
              n218 = Match Pattern(string=w347, regular expression=w346) -> (offset past match=w345:i32)  [unwired: 1 in, 3 out]
              n219 = Greater Or Equal To 0?(x=w345) -> (x >= 0?=w344:bool)
            }
            n220 = case shown="1" w327 {
              tunnel: w326 -> [_ w336 w342]
              tunnel: cluster{"Action":string, "Data":variant} {"Action"="ProjListToActList", "Data"=variant} ("element") -> [_ w331 w337]
              frame Default {
              }
              frame 0 {
                n221 = control-ref of="VirbrationProjectList"() -> (w334:refnum<vi>)
                n222 = control-ref of="VirbList"() -> (w333:refnum<vi>)
                n223 = Bundle("VirbrationProjectList"=w334, "VirbList"=w333) -> (w332:T17)  [unwired: 1 in]
                n224 = Bundle By Name(cluster=w331, "Data"=w332) -> (w335:cluster{"Action":string, "Data":variant})
                n225 = Enqueue Element(queue=w336, element=w335) -> ()  [unwired: 2 in, 3 out]
              }
              frame 1 {
                n226 = control-ref of="IOList"() -> (w338:refnum<vi>)
                n227 = control-ref of="IOProjectList"() -> (w339:refnum<vi>)
                n228 = Bundle("IOProjectList"=w339, "IOList"=w338) -> (w340:T18)  [unwired: 1 in]
                n229 = Bundle By Name(cluster=w337, "Data"=w340) -> (w341:cluster{"Action":string, "Data":variant})
                n230 = Enqueue Element(queue=w342, element=w341) -> ()  [unwired: 2 in, 3 out]
              }
            }
          }
          event Value Change {
            n231 = event-data() -> ("CtlRef"=w349:refnum<vi>)  [unwired: 1 in, 5 out]
            n232 = property class="Bool"(reference=w349) -> ("Label.Text"=w353:string)  [unwired: 1 in, 2 out]
            n233 = for {
              tunnel: w353 -> [w370]
              tunnel: string[] ["Virb", "IO", "None"] -> [w369] mode=indexing
              tunnel: [w366] -> w352
              i -> [w366]
              stop <- w367 stop-if-true
              n234 = Match Pattern(string=w370, regular expression=w369) -> (offset past match=w368:i32)  [unwired: 1 in, 3 out]
              n235 = Greater Or Equal To 0?(x=w368) -> (x >= 0?=w367:bool)
            }
            n236 = case shown="1" w352 {
              tunnel: w350 -> [_ w359 w365]
              tunnel: cluster{"Action":string, "Data":variant} {"Action"="RemoveListAct", "Data"=variant} ("element") -> [_ w354 w360]
              frame Default {
              }
              frame 0 {
                n237 = control-ref of="VirbrationProjectList"() -> (w357:refnum<vi>)
                n238 = control-ref of="VirbList"() -> (w356:refnum<vi>)
                n239 = Bundle("VirbrationProjectList"=w357, "VirbList"=w356) -> (w355:T17)  [unwired: 1 in]
                n240 = Bundle By Name(cluster=w354, "Data"=w355) -> (w358:cluster{"Action":string, "Data":variant})
                n241 = Enqueue Element(queue=w359, element=w358) -> ()  [unwired: 2 in, 3 out]
              }
              frame 1 {
                n242 = control-ref of="IOList"() -> (w361:refnum<vi>)
                n243 = control-ref of="IOProjectList"() -> (w362:refnum<vi>)
                n244 = Bundle("IOProjectList"=w362, "IOList"=w361) -> (w363:T18)  [unwired: 1 in]
                n245 = Bundle By Name(cluster=w360, "Data"=w363) -> (w364:cluster{"Action":string, "Data":variant})
                n246 = Enqueue Element(queue=w365, element=w364) -> ()  [unwired: 2 in, 3 out]
              }
            }
          }
          event "Btn_Save": Value Change {
            n247 = event-data() -> ()  [unwired: 1 in, 6 out]
            n248 = property on="ActionTable" class="MCListbox (strict)"() -> ("ItemNames"=w373:string[][])  [unwired: 2 in, 2 out]
            n249 = property on="VisionTable" class="MCListbox (strict)"() -> ("ItemNames"=w371:string[][])  [unwired: 2 in, 2 out]
            n250 = Build Array (concatenate)(w371, w373) -> (w372:string[][])
            n251 = call "Process List FGV.vi"("TableIn"=w372, "Action"=T10."WrteAll") -> ("error out"=w377:errorcluster)  [unwired: 11 in, 2 out]
            n252 = call "Process List FGV.vi"("Action"=T10."Save", "error in"=w377) -> ("error out"=w374:errorcluster)  [unwired: 11 in, 2 out]
            n253 = call "Request UI.vi"("error in (no error)"=w374, "Wait Reply"=FALSE, "Data"=cluster{"Action":string, "Data":variant} {"Action"="ProjectToUI", "Data"=variant}) -> ()  [unwired: 7 in, 2 out]
          }
          event Value Change {
            n254 = event-data() -> ()  [unwired: 1 in, 6 out]
            n255 = Enqueue Element(queue=w381, element=cluster{"Action":string, "Data":variant} {"Action"="InsertToList", "Data"=variant}) -> ()  [unwired: 2 in, 3 out]
          }
          event Value Change {
            # "RemoveFroimList"
            n256 = event-data() -> ()  [unwired: 1 in, 6 out]
            n257 = for {
              tunnel: w383 -> [w385]
              tunnel: cluster{"Action":string, "Data":variant}[] [{"Action"="CheckRemoveItemName", "Data"=variant}, {"Action"="RemoveFroimList", "Data"=variant}] -> [w384] mode=indexing
              n258 = Enqueue Element(queue=w385, element=w384) -> ()  [unwired: 2 in, 3 out]
            }
          }
          event Value Change {
            n259 = event-data() -> ()  [unwired: 1 in, 6 out]
          }
          event Value Change {
            n260 = event-data() -> ()  [unwired: 1 in, 2 out]
          }
          event "VisionProjectList": Value Change {
            n261 = event-data() -> ("NewVal"=w389:u16)  [unwired: 1 in, 5 out]
            n262 = Decrement(x=w389) -> (x-1=w388:u16)
            n263 = call "Parsing Vision Result For Set.vi"("VisionProject"=w388) -> ("Dataout"=w386:string, "DataoutName"=w387:string)  [unwired: 9 in]
            n264 = local write "DataOutName"(w387) -> ()
            n265 = local write "DataOutResult"(w386) -> ()
          }
          event "UpdateActLisrVir": Value Change {
            n266 = event-data() -> ()  [unwired: 1 in, 6 out]
            n267 = Enqueue Element(queue=w391, element=cluster{"Action":string, "Data":variant} {"Action"="SetToActlist", "Data"=variant}) -> ()  [unwired: 2 in, 3 out]
          }
        }
      }
      n268 = Enqueue Element(queue=w15, element=cluster{"Action":string, "Data":variant} {"Action"="exit", "Data"=variant}) -> ()  [unwired: 2 in, 3 out]
    }
  }
